vi "ge_TC Table Data.vi"(11 "Thrmcpl Type":u16) -> (3 "Type Min/Max":dbl[](array[numeric]))   [LabVIEW 2018]
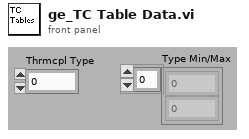
[diagram p1: front panel]
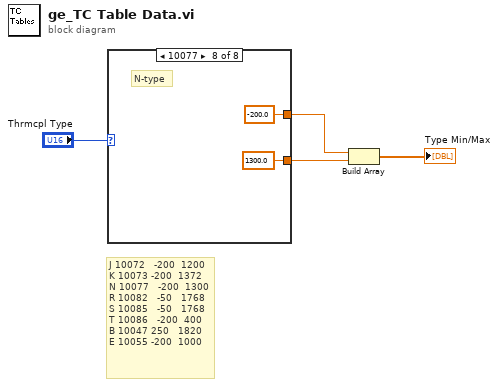
[diagram p0: block diagram]
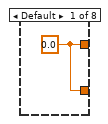
[diagram p2: hidden frame]
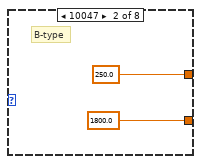
[diagram p3: hidden frame]
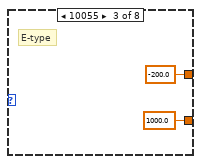
[diagram p4: hidden frame]
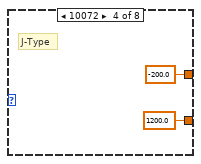
[diagram p5: hidden frame]
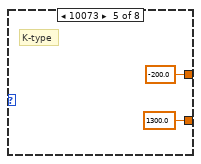
[diagram p6: hidden frame]
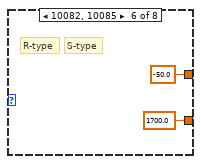
[diagram p7: hidden frame]
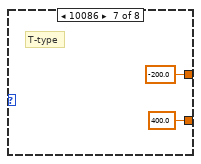
[diagram p8: hidden frame]
diagram:
  # "J\t10072   -200  1200\nK\t10073\t-200  1372\nN\t10077   -200  1300\nR\t10082   -50   1768\nS\t10085   -50   1768\nT\t10086   -200  400\nB\t10047\t250   1820\t\t\nE\t10055\t-200  1000"
  n1 = case shown="10077" "Thrmcpl Type" {
    tunnel: [w5 250.0 -200.0 -200.0 -200.0 -50.0 -200.0 -200.0] -> w2
    tunnel: [w5 1800.0 1000.0 1200.0 1300.0 1700.0 400.0 1300.0] -> w1
    frame Default {
      w5 = 0.0
    }
    frame 10047 {
      # "B-type"
    }
    frame 10055 {
      # "E-type"
    }
    frame 10072 {
      # "J-Type"
    }
    frame 10073 {
      # "K-type"
    }
    frame 10082, 10085 {
      # "S-type"
      # "R-type"
    }
    frame 10086 {
      # "T-type"
    }
    frame 10077 {
      # "N-type"
    }
  }
  n2 = Build Array(w2, w1) -> (→"Type Min/Max":dbl[])
